vi "lB 2.vi"() -> ()   [LabVIEW 2020]
panel:
  out "Array":dbl[](array[numeric])
  in  "Numeric":dbl
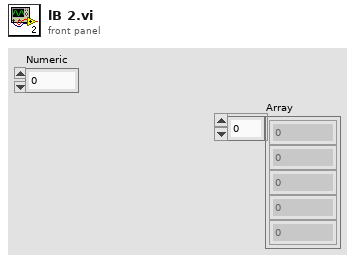
[diagram p1: front panel]
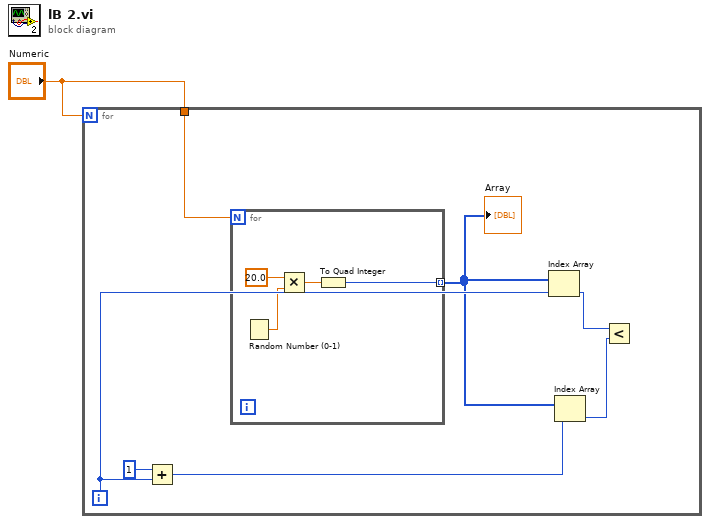
[diagram p0: block diagram]
diagram:
  n1 = for {
    N: "Numeric" -> [_]
    tunnel: "Numeric" -> [w8]
    i -> [w6]
    n2 = Add(x=1, y=w6) -> (x+y=w4:i32)
    n3 = for {
      N: w8 -> [_]
      tunnel: [w9] -> w2 mode=indexing
      n4 = Random Number (0-1)() -> (number: 0 to 1=w11:dbl)
      n5 = Multiply(x=20.0, y=w11) -> (x*y=w10:dbl)
      n6 = To Quad Integer(1:w10) -> (0:w9:i64)
    }
    "Array" <- w2
    n7 = Index Array(array=w2, index=w6) -> (element=w7:i64)
    n8 = Index Array(array=w2, index=w4) -> (element=w3:i64)
    n9 = Less?(x=w7, y=w3) -> ()  [unwired: 1 out]
  }
